vi "calculate scale.vi"(4 "Scaling in":T1={"conversion matrix"=[[0.0, 0.0], [0.0, 0.0], [0.0, 0.0], [0.0, 0.0], [0.0, 0.0], [0.0, 0.0]], "units"="", "name"="", "scale type"=enum."Volts", "offset (volts)"=0.0, "second channel"=0, "correspondence table"=[], "offset (physical units)"=0.0, "pH scale"={"Buffers"=[], "Temperature"=0.0}, "D.O."={"Temperature"=0.0, "K"=0.0, "barometric pressure"=0.0}} {"D.O."."K" format="%.6f"; "D.O."."Temperature" format="%.2f"; "pH scale"."Buffers"."V/T" format="%.5f"; "pH scale"."Buffers"."Buffer" format="%.2f"; "pH scale"."Temperature" format="%.2f"; "offset (physical units)" format="%.5f"; "correspondence table"."volts" format="%.4f"; "correspondence table"."physical units" format="%.4f"; "second channel" min=-1; "offset (volts)" format="%.5f"; "conversion matrix" format="%.4e"}, 5 "reset":bool, 7 "polynomial order":i32=2, 8 "data points to acquire":u32=1000 min=1, 9 "volts array":sgl[](array[numeric]) format="%.5f", 10 "Position":dbl format="%.2f") -> (1 "Scaling out":T1={"conversion matrix"=[[0.0, 0.0], [0.0, 0.0], [0.0, 0.0], [0.0, 0.0], [0.0, 0.0], [0.0, 0.0]], "units"="", "name"="", "scale type"=enum."Volts", "offset (volts)"=0.0, "second channel"=0, "correspondence table"=[], "offset (physical units)"=0.0, "pH scale"={"Buffers"=[], "Temperature"=0.0}, "D.O."={"Temperature"=0.0, "K"=0.0, "barometric pressure"=0.0}} {"D.O."."K" format="%.6f"; "D.O."."Temperature" format="%.2f"; "pH scale"."Buffers"."V/T" format="%.5f"; "pH scale"."Buffers"."Buffer" format="%.2f"; "pH scale"."Temperature" format="%.2f"; "offset (physical units)" format="%.5f"; "correspondence table"."volts" format="%.4f"; "correspondence table"."physical units" format="%.4f"; "second channel" min=-1; "offset (volts)" format="%.5f"; "conversion matrix" format="%.4e"}, 2 "error graph":cluster{"X array":sgl[], "Y array":dbl[]}[](array[cluster]) {"Y array" format="%.2f"; "X array" format="%.2f"}, 3 "Output Graph":cluster{"X array":sgl[], "Y array":dbl[]}[](array[cluster]) {"Y array" format="%.6f"; "X array" format="%.6f"})   [LabVIEW 2012]
uses:
  conversion.ctl
  DAQ configuration/scale type.ctl
  correspondence table.ctl
  pH/pH scale.ctl
  Dissolved Oxygen/DO scale.ctl
  <vilib>/Analysis/baseanly.llb/Mean (DBL).vi
  <vilib>/Analysis/NI_AALPro.lvlib
  <vilib>/Analysis/NI_AALBase.lvlib
panel:
  # "C"
  # "kPa"
  # "C"
  # "C"
  # "kPa"
  # "C"
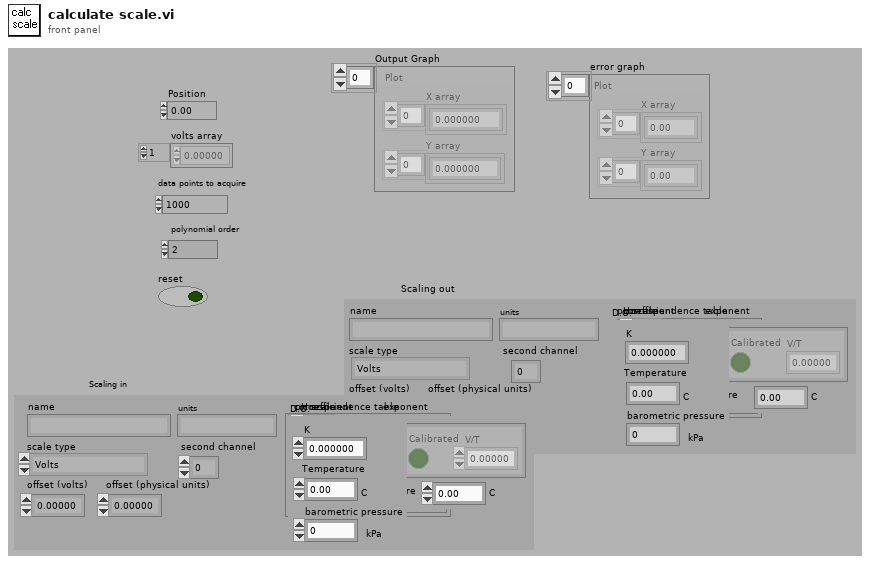
[diagram p1: front panel]
types:
  T1 = typedef "conversion.ctl" = cluster{"conversion matrix":sgl[][], "units":string, "name":string, "scale type":T2, "offset (volts)":dbl, "second channel":i8, "correspondence table":T3, "offset (physical units)":dbl, "pH scale":T4, "D.O.":T5}
  T2 = typedef "scale type.ctl" = enum16{"Volts", "Polynomial", "Correspondence Table", "pH", "Dissolved Oxygen", "Quadratic"}
  T3 = typedef "correspondence table.ctl" = cluster{"physical units":dbl, "volts":dbl}[]
  T4 = typedef "pH scale.ctl" = cluster{"Buffers":cluster{"Buffer":dbl, "Calibrated":bool, "V/T":dbl}[], "Temperature":dbl}
  T5 = typedef "DO scale.ctl" = cluster{"Temperature":dbl, "K":dbl, "barometric pressure":dbl}
  T6 = enum16{"Volts", "Polynomial", "Correspondence Table", "pH", "Dissolved Oxygen"}
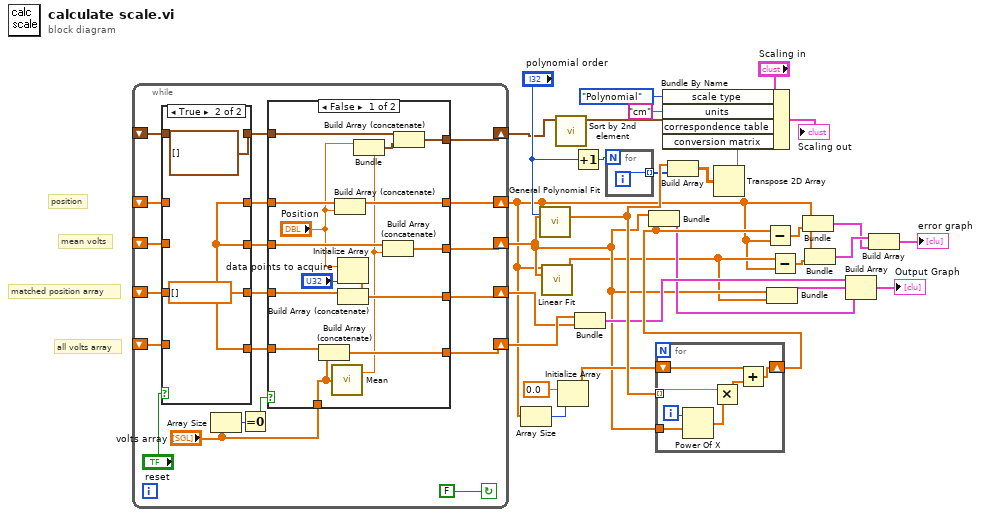
[diagram p0: block diagram]
diagram:
  # "matched position array"
  # "mean volts"
  # "all volts array"
  # "position"
  n1 = while {
    shift-left: _ -> [w34]
    shift-right: [w36] -> w1
    shift-left: _ -> [w37]
    shift-right: [w39] -> w8
    shift-left: _ -> [w42]
    shift-right: [w40] -> w5
    shift-left: _ -> [w43]
    shift-right: [w48] -> w19
    shift-left: _ -> [w45]
    shift-right: [w49] -> w18
    stop <- FALSE continue-if-true
    n2 = case shown="True" "reset" {
      tunnel: [w76 w78] -> w46
      tunnel: w45 -> [w76 _]
      tunnel: [w75 w78] -> w44
      tunnel: w43 -> [w75 _]
      tunnel: w42 -> [w74 _]
      tunnel: [w74 w78] -> w41
      tunnel: [w73 w78] -> w38
      tunnel: w37 -> [w73 _]
      tunnel: [w72 cluster{"Position":sgl, "mean":dbl}[] []] -> w35
      tunnel: w34 -> [w72 _]
      frame False {
      }
      frame True {
        w78 = sgl[] []
      }
    }
    n3 = Array Size(array="volts array") -> (size(s)=w32:i32)
    n4 = Equal To 0?(x=w32) -> (x = 0?=w31:bool)
    n5 = case shown="False" w31 {
      tunnel: [w66 w68] -> w49
      tunnel: [w65 w67] -> w48
      tunnel: w46 -> [w64 w68]
      tunnel: w44 -> [w63 w67]
      tunnel: "volts array" -> [w60 _]
      tunnel: w41 -> [w59 w70]
      tunnel: [w58 w70] -> w40
      tunnel: [w57 w69] -> w39
      tunnel: w38 -> [w56 w69]
      tunnel: [w53 w71] -> w36
      tunnel: w35 -> [w52 w71]
      frame False {
        n6 = Build Array (concatenate)(w63, w60) -> (w65:sgl[])
        n7 = call-poly <vilib>:"Mean.vi"("X"=w60) -> ("mean"=w51:dbl)  [unwired: 1 out]
        n8 = Build Array (concatenate)(w59, "Position") -> (w58:dbl[])
        n9 = Initialize Array("Position", "data points to acquire") -> (w61:dbl[])
        n10 = Build Array (concatenate)(w64, w61) -> (w66:dbl[])
        n11 = Bundle("Position"="Position", "mean"=w51) -> (w54:cluster{"Position":dbl, "mean":dbl})  [unwired: 1 in]
        n12 = Build Array (concatenate)(w56, w51) -> (w57:dbl[])
        n13 = Build Array (concatenate)(w52, w54) -> (w53:cluster{"Position":dbl, "mean":dbl}[])
      }
      frame True {
      }
    }
  }
  n14 = Array Size(array=w5) -> (size(s)=w4:i32)
  n15 = call <vilib>:"General Polynomial Fit.vi"("Y"=w5, "polynomial order"="polynomial order", "X"=w8) -> ("Polynomial Coefficients"=w21:dbl[])  [unwired: 9 in, 3 out]
  n16 = call <vilib>:"Linear Fit.vi"("Y"=w5, "X"=w8) -> ("Best Linear Fit"=w7:dbl[])  [unwired: 9 in, 4 out]
  n17 = call "Sort by 2nd element.vi"("correspondence table in"=w1) -> ("correspondence table out"=w2:T3)  [unwired: 9 in]
  n18 = Initialize Array(0.0 ("Element Data"), w4) -> (w16:dbl[])
  n19 = Increment(x="polynomial order") -> (x+1=w28:i32)
  n20 = Bundle(w19, w18) -> (w10:cluster{sgl[], dbl[]})  [unwired: 1 in]
  n21 = for {
    N: w28 -> [_]
    tunnel: [w79] -> w20 mode=indexing
    i -> [w79]
  }
  n22 = for {
    tunnel: w21 -> [w86] mode=indexing
    tunnel: w8 -> [w81]
    shift-right: [w84] -> w22
    shift-left: w16 -> [w83]
    i -> [w80]
    n23 = Power Of X(1:w81, 2:w80) -> (0:w85:dbl[])
    n24 = Multiply(x=w86, y=w85) -> (x*y=w82:dbl[])
    n25 = Add(x=w83, y=w82) -> (x+y=w84:dbl[])
  }
  n26 = Bundle(w8, w22) -> (w9:cluster{dbl[], dbl[]})  [unwired: 1 in]
  n27 = Build Array(w21, w20) -> (w27:dbl[][])
  n28 = Transpose 2D Array(2D array=w27) -> (transposed array=w26:dbl[][])
  n29 = Bundle By Name(cluster="Scaling in", "scale type"=T6."Polynomial", "units"="cm", "correspondence table"=w2, "conversion matrix"=w26) -> (→"Scaling out":T1)
  n30 = Subtract(x=w22, y=w5) -> (x-y=w15:dbl[])
  n31 = Bundle(w8, "Best Linear Fit"=w7) -> (w6:cluster{dbl[], "Best Linear Fit":dbl[]})  [unwired: 1 in]
  n32 = Subtract(x=w7, y=w5) -> (x-y=w14:dbl[])
  n33 = Bundle(w5, w15) -> (w11:cluster{dbl[], dbl[]})  [unwired: 1 in]
  n34 = Bundle(w5, w14) -> (w12:cluster{dbl[], dbl[]})  [unwired: 1 in]
  n35 = Build Array(w10, w6, w9) -> (→"Output Graph":cluster{dbl[], "Best Linear Fit":dbl[]}[])
  n36 = Build Array(w12, w11) -> (→"error graph":cluster{dbl[], dbl[]}[])
